vi "Close Device.vi"(8 "error in (no error)":errorcluster, 11 "Simulated-Topas in":refnum<class "Simulated-Topas.lvclass">) -> (0 "error out":errorcluster, 3 "Simulated-Topas out":refnum<class "Simulated-Topas.lvclass">)   [LabVIEW 2020, in "Simulated-Topas.lvclass"]
uses:
  Simulated-Topas.lvclass
  Abstract Topas/Abstract Topas.lvclass
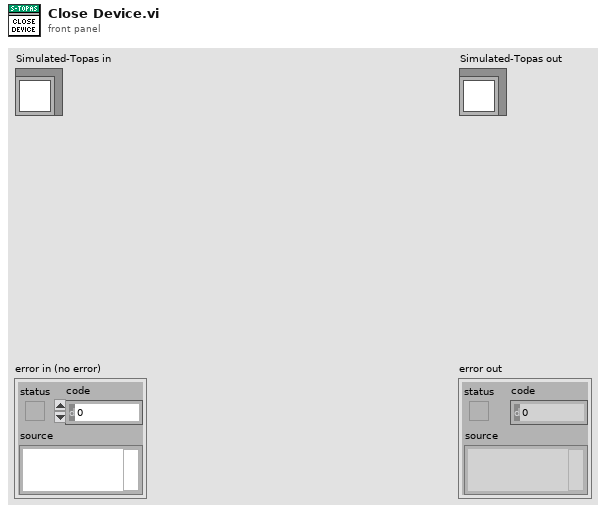
[diagram p1: front panel]
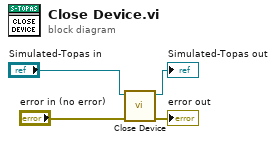
[diagram p0: block diagram]
diagram:
  n1 = call-parent "Close Device.vi"("error in (no error)"="error in (no error)", "Abstract Topas in"="Simulated-Topas in") -> ("error out"=→"error out":errorcluster, "Abstract Topas out"=→"Simulated-Topas out":refnum<class "Simulated-Topas.lvclass">)  [unwired: 8 in]
